vi "First Step.vi"(8 "error in (no error)":errorcluster, 11 "Function Gen Scan.lvclass in":refnum<class "Function Gen Scan.lvclass">) -> (0 "error out":errorcluster, 2 "Current Position":dbl, 3 "Function Gen Scan.lvclass out":refnum<class "Function Gen Scan.lvclass">)   [LabVIEW 2017, in "Function Gen Scan.lvclass"]
doc: "(Dynamic) Reset the instrument and prepare to scan. Goto step #0 - the first step. If desired, the scanner may do this in a different way than usual (i.e. by preparing to move a long distance, or reset to home position.)"
uses:
  Function Gen Scan.lvclass
  Function Gen Scan.lvclass/Function Gen Scan.ctl
  Scanner/Scanner.lvclass
  Instruments/Utility Classes/Scannable/Scannable.lvclass
  Instruments/Function Generator/Tektronix AFG 3000 Series/Tektronix AFG 3000 Series.lvlib
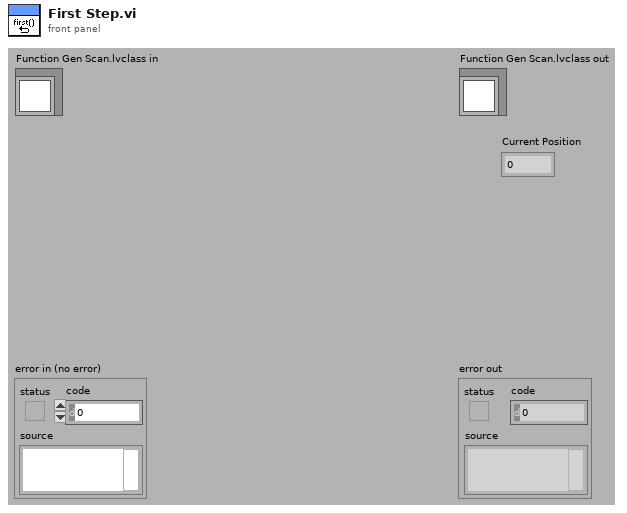
[diagram p1: front panel]
types:
  T1 = typedef "Channel.ctl" = u16
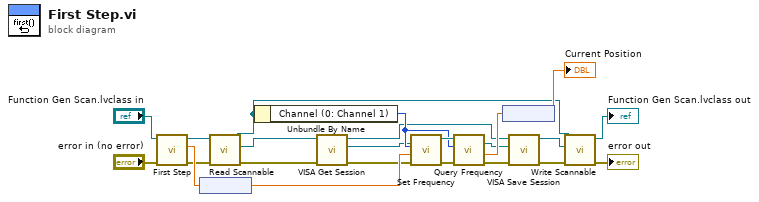
[diagram p0: block diagram]
diagram:
  n1 = call-parent "First Step.vi"("error in (no error)"="error in (no error)", "Scanner.lvclass in"="Function Gen Scan.lvclass in") -> ("error out"=w13:errorcluster, "Current Position"=w21:dbl, "Scanner.lvclass out"=w14:refnum<class "Function Gen Scan.lvclass">)  [unwired: 7 out]
  n2 = node(w21) -> (w20:dbl[unit])
  n3 = call-dynamic "Read Scannable.vi"("error in (no error)"=w13, "Scanner.lvclass in"=w14) -> ("error out"=w11:errorcluster, "Scannable.lvclass"=w12:refnum<class "Scannable.lvclass">, "Scanner.lvclass out"=w2:refnum<class "Function Gen Scan.lvclass">)  [unwired: 7 out]
  n4 = Unbundle By Name(w2) -> ("Channel (0: Channel 1)"=w17:T1)
  n5 = call-dynamic "VISA Get Session.vi"("error in (no error)"=w11, "Instrument.lvclass in"=w12) -> ("error out"=w10:errorcluster, "VISA Resource Name"=w9:refnum<visa-resource-name>, "Instrument.lvclass out"=w7:refnum<class "Scannable.lvclass">)  [unwired: 7 out]
  n6 = call "Set Frequency.vi"("error in (no error)"=w10, "frequency"=w20, "Channel (0: Channel 1)"=w17, "VISA resource name"=w9) -> ("error out"=w19:errorcluster, "VISA resource name out"=w18:refnum<visa-resource-name>)  [unwired: 6 out]
  n7 = call "Query Frequency.vi"("error in (no error)"=w19, "Channel (0: Channel 1)"=w17, "VISA resource name"=w18) -> ("error out"=w8:errorcluster, "frequency"=w16:dbl[unit], "VISA resource name out"=w6:refnum<visa-resource-name>)  [unwired: 6 out]
  n8 = node(w16) -> (→"Current Position":dbl)
  n9 = call-dynamic "VISA Save Session.vi"("error in (no error)"=w8, "VISA Resource Name"=w6, "Instrument.lvclass in"=w7) -> ("error out"=w5:errorcluster, "Instrument.lvclass out"=w1:refnum<class "Scannable.lvclass">)  [unwired: 7 out]
  n10 = call-dynamic "Write Scannable.vi"("error in (no error)"=w5, "Scannable.lvclass"=w1, "Scanner.lvclass in"=w2) -> ("error out"=→"error out":errorcluster, "Scanner.lvclass out"=→"Function Gen Scan.lvclass out":refnum<class "Function Gen Scan.lvclass">)  [unwired: 7 out]
